vi "控制命令区.vi"(10 "控制命令参数":u16[](array[numeric]), 11 "控制命令":u16(ring) items=["启动测量"=1, "标样测量"=2, "零点核查"=3, "跨度核查"=4, "空白测试"=5, "平行样测试"=6, "加标回收"=7, "空白测试"=8, "标样校准"=9, "初始化（清洗）"=10, "停止测试"=11, "仪器重启"=12, "校时"=13, "模式设置"=14, "测量间隔设置"=15]) -> (3 "控制命令":u16[](array[numeric]))   [LabVIEW 2016, in "氨氮.lvlib"]
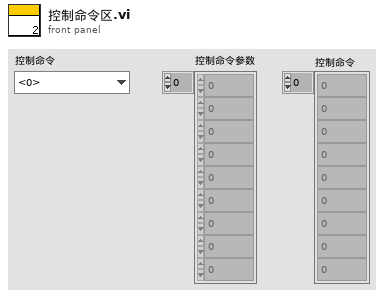
[diagram p1: front panel]
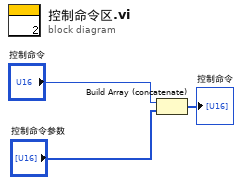
[diagram p0: block diagram]
diagram:
  n1 = Build Array (concatenate)("控制命令", "控制命令参数") -> (→"控制命令":u16[])
